vi "Actor Core.vi"(8 "error in":errorcluster, 11 "Nested in":refnum<class "Manejador de Turnos.lvclass">) -> (0 "error out":errorcluster, 3 "Actor out":refnum<class "Actor.lvclass">)   [LabVIEW 2020, in "Manejador de Turnos.lvlib" / "Manejador de Turnos.lvclass"]
doc: "(<B>Filename</B>: Actor Framework.lvlib:Actor.lvclass:Actor Core.vi)\n\nReceives messages to the actor, reacts to them, and initiates any error handling that may shut the actor down.\n\nDescendant classes may override this VI to append parallel tasks for the actor to complete while it handles messages. Overrides use the Call Parent Method node."
uses:
  Manejador de Turnos.lvclass
  <vilib>/ActorFramework/Actor/Actor.lvclass
  <vilib>/ActorFramework/Stop Msg/Stop Msg.lvclass
  Manejador de Turnos Messages/Set the Turn Msg/Set the Turn Msg.lvclass
panel:
  in  "Selector":dbl
  in  "Cancel Button":bool
  out "Item Names":string[][](array[string])
  out "Column Header Strings[]":string[](array[string])
  out "Multicolumn Listbox":i32(listbox)
  out "Encerado":bool
  out "Lavado\nMotor":bool
  out "Aspirado":bool
  out "Secado":bool
  out "Enjuagado":bool
  out "Enjabonado":bool
  out "Mojado":bool
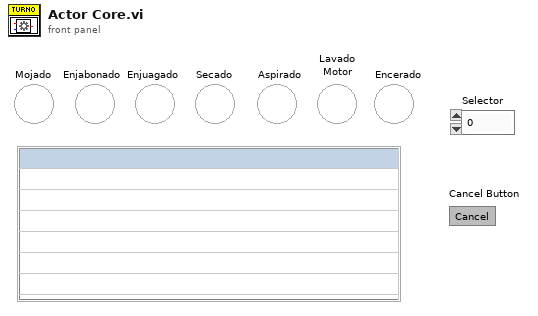
[diagram p1: front panel]
types:
  T1 = cluster{"Stop":refnum<user-event>, "Multicolumn Listbox":refnum<user-event>, "Item Names":refnum<user-event>, "Column Header Strings[]":refnum<user-event>}
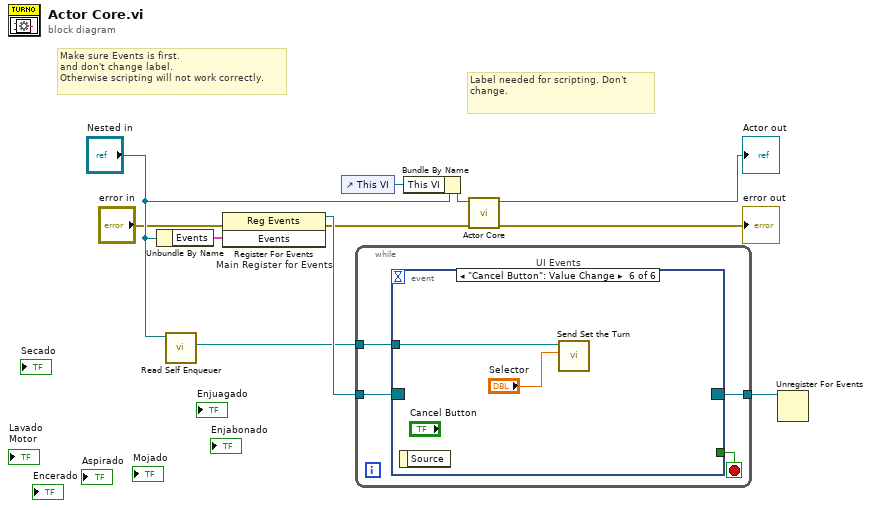
[diagram p0: block diagram]
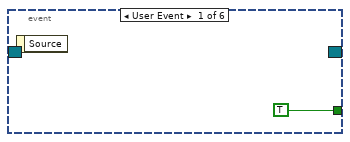
[diagram p2: hidden frame]
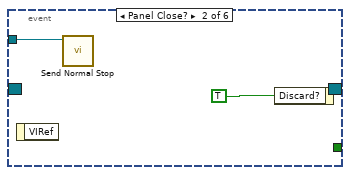
[diagram p3: hidden frame]
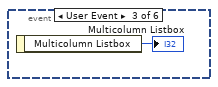
[diagram p4: hidden frame]
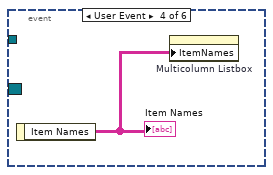
[diagram p5: hidden frame]
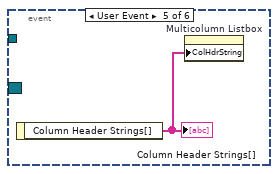
[diagram p6: hidden frame]
diagram:
  # "Label needed for scripting. Don't change."
  # "Make sure Events is first.\nand don't change label.\nOtherwise scripting will not work correctly."
  n1 = Unbundle By Name("Nested in") -> ("Events"=w8:T1)
  n2 = call <vilib>:"Read Self Enqueuer.vi"("Actor"="Nested in") -> ("Self Enqueuer"=w5:refnum<class "Message Enqueuer.lvclass">)  [unwired: 10 in]
  n3 = register-events "Main Register for Events"(error in="error in", w8) -> (reference out=w9:refnum<event-registration>, error out=w3:errorcluster)  [unwired: 1 in]
  n4 = control-ref of="This VI"() -> (w1:refnum<vi>)
  n5 = while {
    tunnel: w9 -> [w15]
    tunnel: [w13] -> w7
    tunnel: w5 -> [w12]
    stop <- w14 stop-if-true
    n6 = event "UI Events" shown="[5] \"Cancel Button\": Value Change" {
      selector: w15 -> [_ _ _ _ _ _]
      dyn-events: [_ _ _ _ _ _] -> w13
      timeout: _ -> [_ _ _ _ _ _]
      tunnel: [TRUE _ _ _ _ _] -> w14
      tunnel: w12 -> [_ w17 _ _ _ w23]
      event User Event {
        n7 = event-data() -> ()  [unwired: 1 in, 1 out]
      }
      event Panel Close? {
        n8 = event-data() -> ()  [unwired: 1 in, 1 out]
        n9 = call <vilib>:"Send Normal Stop.vi"("Message Enqueuer"=w17) -> ()  [unwired: 10 in, 1 out]
        n10 = event-data("Discard?"=TRUE) -> ()  [unwired: 1 in, 1 out]
      }
      event User Event {
        n11 = event-data() -> ("Multicolumn Listbox"=→"Multicolumn Listbox":i32)  [unwired: 1 in]
      }
      event User Event {
        n12 = event-data() -> ("Item Names"=w20:string[][])  [unwired: 1 in]
        "Item Names" <- w20
        n13 = property on="Multicolumn Listbox" class="MCListbox (strict)"("ItemNames"=w20) -> ()  [unwired: 2 in, 2 out]
      }
      event User Event {
        n14 = event-data() -> ("Column Header Strings[]"=w21:string[])  [unwired: 1 in]
        "Column Header Strings[]" <- w21
        n15 = property on="Multicolumn Listbox" class="MCListbox (strict)"("ColHdrString"=w21) -> ()  [unwired: 2 in, 2 out]
      }
      event "Cancel Button": Value Change {
        n16 = event-data() -> ()  [unwired: 1 in, 1 out]
        n17 = call "Send Set the Turn.vi"("Selector"="Selector", "Message Enqueuer"=w23) -> ()  [unwired: 8 in, 2 out]
      }
    }
  }
  n18 = Bundle By Name(cluster="Nested in", "This VI"=w1) -> (w2:refnum<class "Manejador de Turnos.lvclass">)
  n19 = call-parent "Actor Core.vi"("error in"=w3, "Actor in"=w2) -> ("error out"=→"error out":errorcluster, "Actor out"=→"Actor out":refnum<class "Actor.lvclass">)  [unwired: 8 in]
  n20 = Unregister For Events(event registration refnum=w7) -> ()  [unwired: 1 in, 1 out]
